vi "2.vi"() -> ()   [LabVIEW 2015]
panel:
  out "Array 2":i32[](array[numeric])=[4, 6, 10]
  in  "Array":dbl[](array[numeric])=[1.0, 10.0, 0.0, -8.0, 14.0, 2.0, 14.0, 3.0, -5.0, -1.0, 14.0, -9.0]
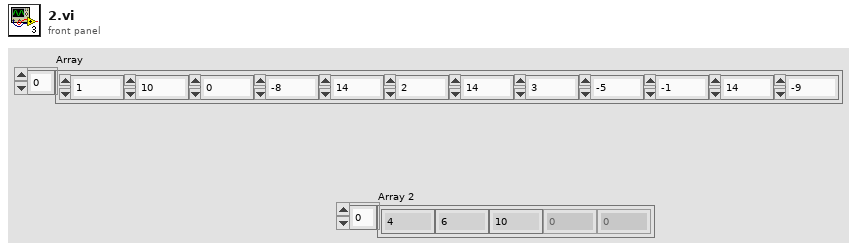
[diagram p1: front panel]
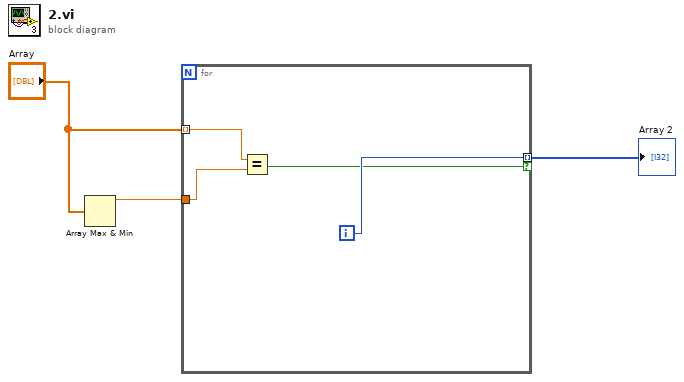
[diagram p0: block diagram]
diagram:
  n1 = Array Max & Min(array="Array") -> (max value=w3:dbl)  [unwired: 3 out]
  n2 = for {
    tunnel: w3 -> [w7]
    tunnel: "Array" -> [w6] mode=indexing
    tunnel: [w5] -> w1 mode=indexing if=w4
    i -> [w5]
    n3 = Equal?(x=w6, y=w7) -> (x = y?=w4:bool)
  }
  "Array 2" <- w1
